vi "AM(Sub).vi"(6 "Time (s)":i32=10, 7 "Modulation Index":dbl=1000.0, 8 "Sample":i32=10000, 9 "Modulated Frequency":dbl=200.0, 10 "Carrier Frequency":dbl=200.0, 11 "File":path) -> (1 "Waveform Graph":waveform(dbl)(graph), 2 "Data":dbl[](array[numeric]))   [LabVIEW 2020]
uses:
  <vilib>/Analysis/NI_AALPro.lvlib
panel:
  in  "Carrier Amplitude":dbl=1.0 format="%0.2f"
  out "Array Size":i32
  out "Data 2":dbl[](array[numeric])
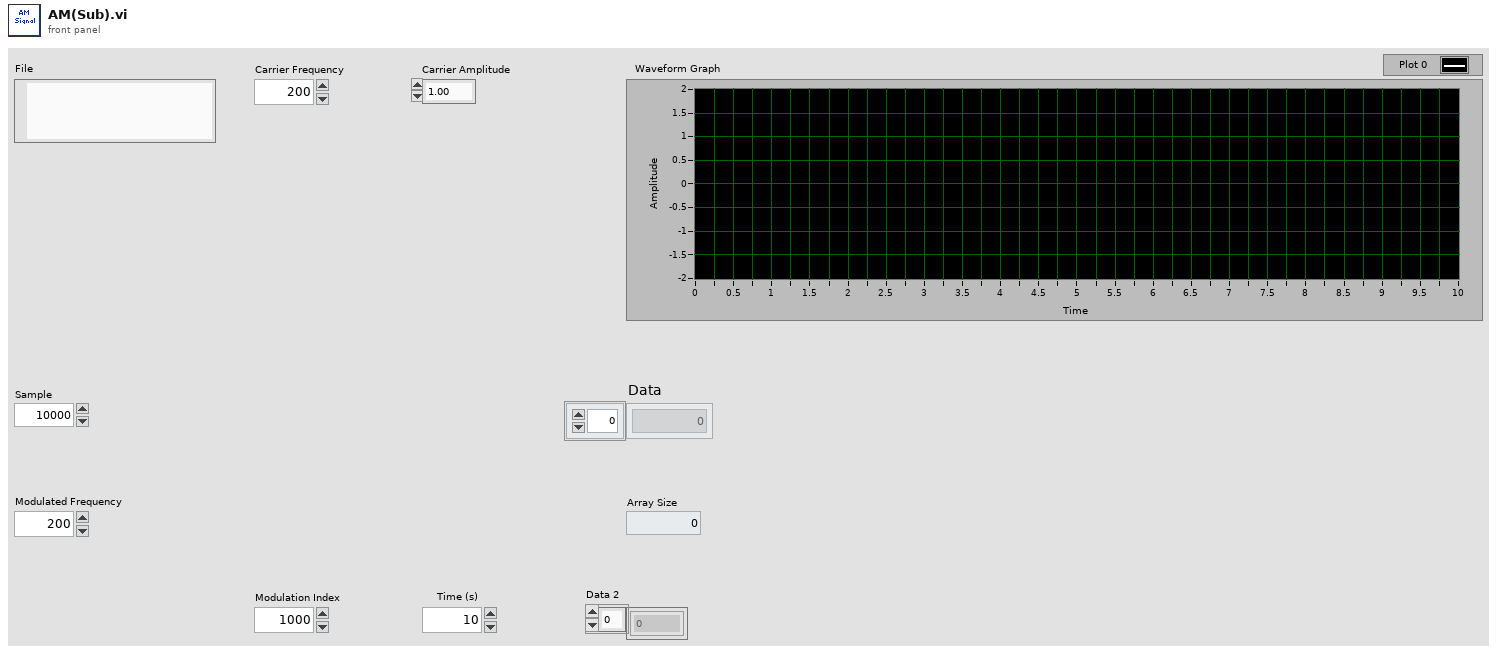
[diagram p1: front panel]
types:
  T1 = enum16{"sine", "cosine", "triangle", "square", "sawtooth", "increasing ramp", "decreasing ramp"}
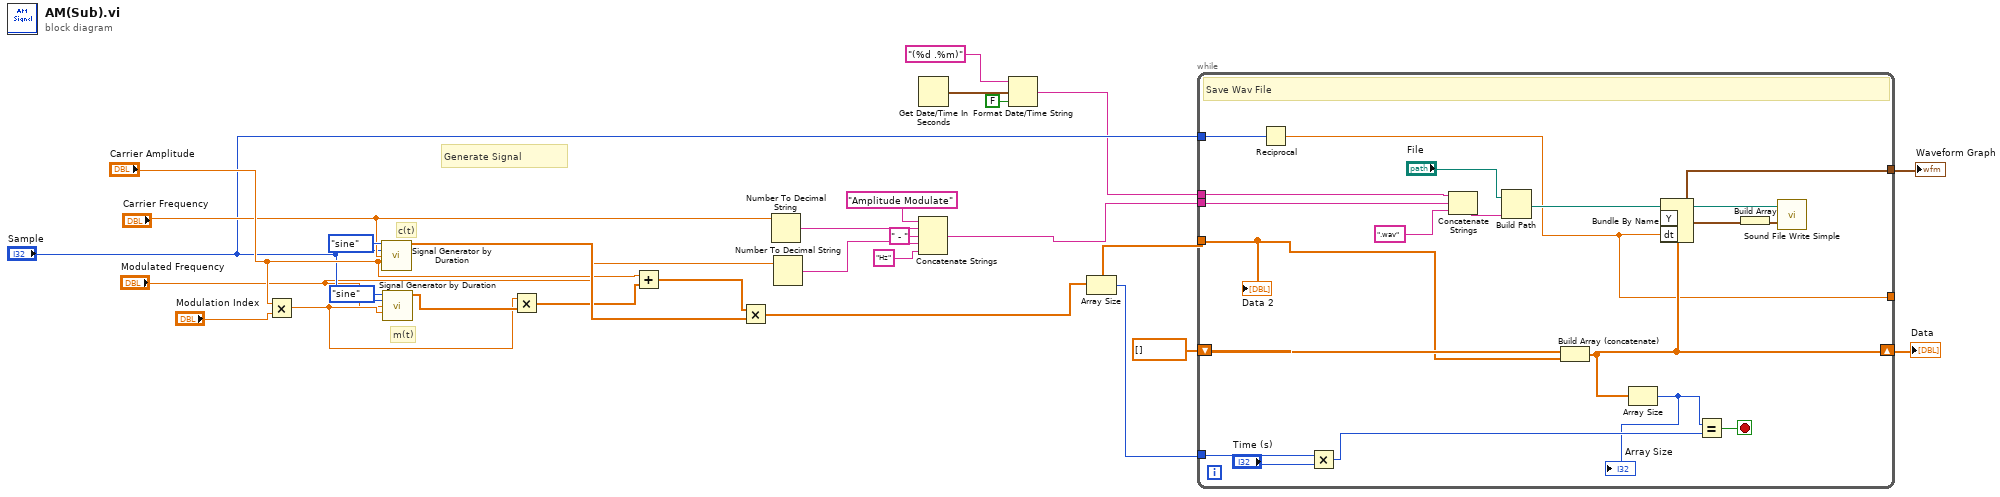
[diagram p0: block diagram]
diagram:
  # "c(t)"
  # "m(t)"
  # "Generate Signal"
  n1 = Multiply(x="Carrier Amplitude", y="Modulation Index") -> (x*y=w21:dbl)
  n2 = call <vilib>:"Signal Generator by Duration.vi"("signal type"=T1."sine", "# of samples"="Sample", "frequency"="Carrier Frequency", "amplitude"="Carrier Amplitude") -> ("signal"=w26:dbl[])  [unwired: 8 in, 3 out]
  n3 = call <vilib>:"Signal Generator by Duration.vi"("signal type"=T1."sine", "# of samples"="Sample", "frequency"="Modulated Frequency", "amplitude"=w21) -> ("signal"=w22:dbl[])  [unwired: 8 in, 3 out]
  n4 = Multiply(x=w21, y=w22) -> (x*y=w24:dbl[])
  n5 = Add(x="Carrier Amplitude", y=w24) -> (x+y=w25:dbl[])
  n6 = Multiply(x=w25, y=w26) -> (x*y=w27:dbl[])
  n7 = Number To Decimal String(number="Carrier Frequency") -> (decimal integer string=w14:string)  [unwired: 1 in]
  n8 = Number To Decimal String(number="Modulated Frequency") -> (decimal integer string=w2:string)  [unwired: 1 in]
  n9 = Concatenate Strings("Amplitude Modulate", w14, " - " ("string"), w2, "Hz" ("string")) -> (w9:string)
  n10 = Get Date/Time In Seconds() -> (seconds since 1Jan1904=w10:timestamp)
  n11 = Format Date/Time String(time format string (%c)="(%d .%m)", seconds (now)=w10, UTC format=FALSE) -> (date/time string=w13:string)
  n12 = Array Size(array=w27) -> (size(s)=w5:i32)
  n13 = while {
    tunnel: "Sample" -> [w45]
    tunnel: w27 -> [w42]
    shift-right: [w41] -> w8
    shift-left: dbl[] [] ("Array") -> [w43]
    tunnel: w5 -> [w37]
    tunnel: [w34] -> _
    tunnel: [w32] -> w7
    tunnel: w9 -> [w31]
    tunnel: w13 -> [w29]
    stop <- w40 stop-if-true
    # "Save Wav File"
    n14 = Reciprocal(x=w45) -> (1/x=w34:dbl)
    n15 = Multiply(x=w37, y="Time (s)") -> (x*y=w39:i32)
    n16 = Concatenate Strings(w29, w31, ".wav") -> (w33:string)
    n17 = Build Path(base path="File", name or relative path=w33) -> (appended path=w44:path)
    n18 = Build Array (concatenate)(w43, w42) -> (w41:dbl[])
    n19 = Array Size(array=w41) -> (size(s)=w38:i32)
    "Array Size" <- w38
    n20 = Bundle By Name("Y"=w41, "dt"=w34) -> (w32:waveform(dbl))  [unwired: 1 in]
    n21 = Equal?(x=w38, y=w39) -> (x = y?=w40:bool)
    n22 = Build Array(w32) -> (w35:waveform(dbl)[])
    n23 = call <vilib>:"Sound File Write Simple.vi"("data"=w35, "path"=w44) -> ()  [unwired: 8 in, 2 out]
    "Data 2" <- w42
  }
  "Data" <- w8
  "Waveform Graph" <- w7
